vi "Recieve Request for Result.vi"(6 "Request time":timestamp, 8 "error in (no error)":errorcluster, 9 "Requestor":string, 10 "Requestee":string, 11 "Measurement Timer in":refnum<class "Measurement Timer.lvclass">) -> (0 "error out":errorcluster, 3 "Measurement Timer out":refnum<class "Measurement Timer.lvclass">)   [LabVIEW 2015, in "Measurement Timer.lvclass"]
uses:
  Measurement Timer.lvclass
  Mag Lab Root/Mag Lab Root.lvclass/Mag Lab Root.ctl
  Mag Lab Result/Mag Lab Result.lvclass
  Timer Parameters.ctl
  Log time.ctl
  <vilib>/ActorFramework/Actor/Actor.lvclass/Actor.ctl
  Measurement Timer.lvclass/Measurement Timer.ctl
  Mag Lab Result/Mag Lab Result.lvclass/Mag Lab Result.ctl
  Mag Lab Root Messages/Recieve Response with Result Msg/Recieve Response with Result Msg.lvclass/Recieve Response with Result Msg.ctl
  <vilib>/ActorFramework/Message Enqueuer/Message Enqueuer.lvclass/Message Enqueuer.ctl
  Mag Lab Result/Write Next time.vi
  Mag Lab Result/Write Group Name.vi
  Mag Lab Result/Write Name.vi
  Mag Lab Result/Write Sets pace.vi
  Mag Lab Result/Write Result time.vi
  <vilib>/ActorFramework/Message Enqueuer/Enqueue.vi
  <vilib>/ActorFramework/Message Priority Queue/Priority Enqueue.vi
  Mag Lab Root Messages/Recieve Response with Result Msg/Recieve Response with Result Msg.lvclass
  Mag Lab Properties/Mag Lab Parameters.lvclass
  Mag Lab Root/Mag Lab Root.lvclass
  <vilib>/ActorFramework/Actor/Actor.lvclass
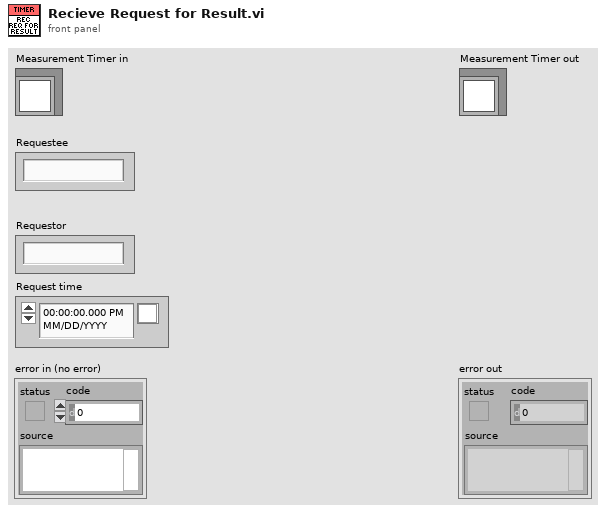
[diagram p1: front panel]
types:
  T1 = typedef "Timer Parameters.ctl" = cluster{"millisecond multiple":u32, "Time reference":T2}
  T2 = typedef "Log time.ctl" = enum16{"Relative", "Absolute", "Do not log"}
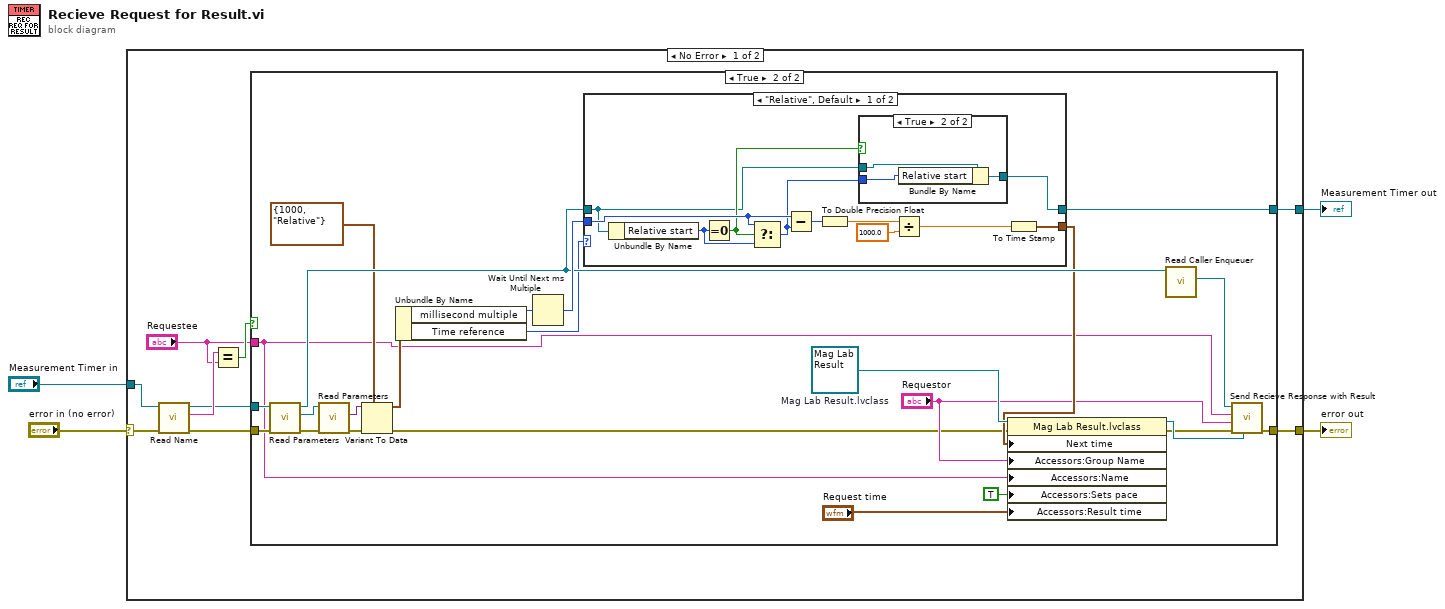
[diagram p0: block diagram]
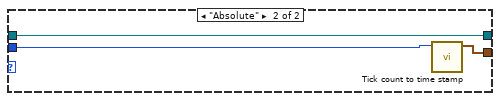
[diagram p4: hidden frame]
diagram:
  n1 = case shown="No Error" "error in (no error)" {
    selector: "error in (no error)" -> [w12 w58]
    tunnel: "Measurement Timer in" -> [w13 w59]
    tunnel: [w7 w59] -> w2
    tunnel: [w6 w58] -> w1
    frame No Error {
      n2 = call "Read Name.vi"("error in (no error)"=w12, "Mag Lab Root in"=w13) -> ("error out"=w5:errorcluster, "Name"=w11:string, "Mag Lab Root out"=w9:refnum<class "Measurement Timer.lvclass">)  [unwired: 7 in]
      n3 = Equal?(x=w11, y="Requestee") -> (x = y?=w10:bool)
      n4 = case shown="True" w10 {
        tunnel: w9 -> [w15 w35]
        tunnel: "Requestee" -> [_ w21]
        tunnel: [w15 w37] -> w7
        tunnel: [w14 w36] -> w6
        tunnel: w5 -> [w14 w33]
        frame False {
        }
        frame True {
          w24 = refnum<class "Mag Lab Result.lvclass"> refnum  # Mag Lab Result.lvclass
          n5 = call-dynamic "Read Parameters.vi"("error in (no error)"=w33, "Mag Lab Root in"=w35) -> ("error out"=w29:errorcluster, "Mag Lab Parameters.lvclass"=w32:refnum<class "Mag Lab Parameters.lvclass">, "Mag Lab Root out"=w34:refnum<class "Measurement Timer.lvclass">)  [unwired: 7 in]
          n6 = call-dynamic "Read Parameters.vi"("error in (no error)"=w29, "Mag Lab Parameters in"=w32) -> ("error out"=w31:errorcluster, "Parameters"=w30:variant)  [unwired: 7 in, 1 out]
          n7 = Variant To Data(error in=w31, type=T1 {"millisecond multiple"=1000, "Time reference"=enum."Relative"} ("Timer Parameters"), Variant=w30) -> (data=w27:T1, error out=w19:errorcluster)
          n8 = Unbundle By Name(w27) -> ("millisecond multiple"=w26:u32, "Time reference"=w25:T2)
          n9 = Wait Until Next ms Multiple(millisecond multiple=w26) -> (millisecond timer value=w39:u32)
          n10 = case shown="\"Relative\", Default" w25 {
            tunnel: w39 -> [w50 w57]
            tunnel: [w49 w56] -> w23
            tunnel: w34 -> [w42 w55]
            tunnel: [w40 w55] -> w37
            frame "Relative", Default {
              n11 = Unbundle By Name(w42) -> ("Relative start"=w44:u64)
              n12 = Equal To 0?(x=w44) -> (x = 0?=w43:bool)
              n13 = Select(t=w50, s=w43, f=w44) -> (s? t:f=w41:u64)
              n14 = Subtract(x=w50, y=w41) -> (x-y=w46:u64)
              n15 = To Double Precision Float(number=w46) -> (double precision float=w48:dbl)
              n16 = case shown="True" w43 {
                tunnel: w42 -> [w51 w54]
                tunnel: w41 -> [_ w53]
                tunnel: [w51 w52] -> w40
                frame False {
                }
                frame True {
                  n17 = Bundle By Name(cluster=w54, "Relative start"=w53) -> (w52:refnum<class "Measurement Timer.lvclass">)
                }
              }
              n18 = Divide(x=w48, y=1000.0) -> (x/y=w45:dbl)
              n19 = To Time Stamp(1:w45) -> (0:w49:timestamp)
            }
            frame "Absolute" {
              n20 = call "Tick count to time stamp.vi"("millisecond timer value in"=w57) -> ("time stamp"=w56:timestamp)  [unwired: 9 in, 1 out]
            }
          }
          n21 = property class="Mag Lab Result.lvclass"(reference=w24, error in=w19, "Next time"=w23, "Accessors:Group Name"="Requestor", "Accessors:Name"=w21, "Accessors:Sets pace"=TRUE ("Sets pace"), "Accessors:Result time"="Request time") -> (reference out=w20:refnum<class "Mag Lab Result.lvclass">, error out=w18:errorcluster)
          n22 = call <vilib>:"Read Caller Enqueuer.vi"("Actor"=w34) -> ("Caller Enqueuer"=w38:refnum<class "Message Enqueuer.lvclass">)  [unwired: 10 in]
          n23 = call "Send Recieve Response with Result.vi"("Result"=w20, "error in (no error)"=w18, "Requestor"="Requestor", "Requestee"=w21, "Message Enqueuer"=w38) -> ("error out"=w36:errorcluster)  [unwired: 5 in, 1 out]
        }
      }
    }
    frame Error {
    }
  }
  "error out" <- w1
  "Measurement Timer out" <- w2
